vi "akcelerometr.vi"() -> ()   [LabVIEW 2014]
doc: "This example demonstrates how to read X, Y, and Z accelerations using the MMA8452 accelerometer."
uses:
  <vilib>/MakerHub/LINX/Public/Utilities/Open Local.vi
  <vilib>/MakerHub/LINX/LMH-LINX.lvlib
panel:
  out "k¹t nachylenia":dbl
  in  "Stop Button":bool
  out "Waveform Chart":T1(graph)
  out "Loop Rate (Hz)":u32
  # "LIS3DH Accelerometer\n\nThis example demonstrates how to read three axis of acceleration from the LIS3DH \\ MMA8452Q accelerometer \n\nInstructions\n1. Select the COM Port associated with the LINX Device.\n2. Select the I2C Channel that the MMA8452Q is connected to.\n3. Click the Run Arrow."
  # "Analog Value"
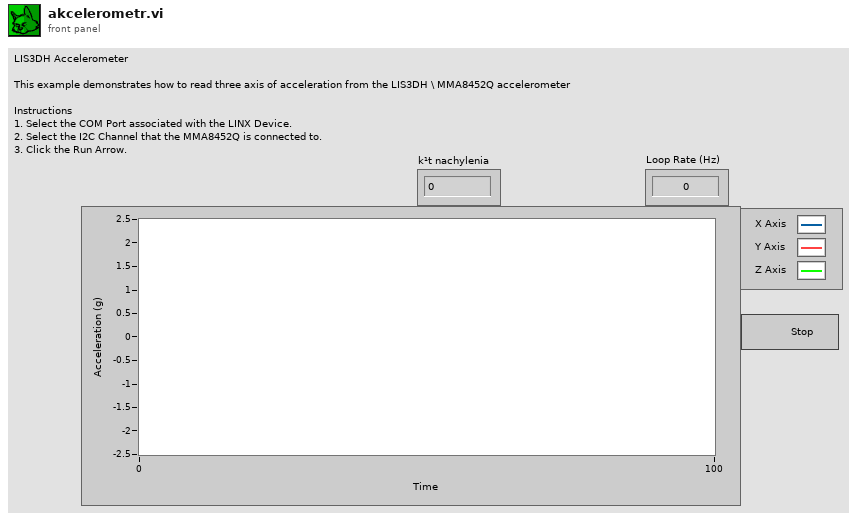
[diagram p1: front panel]
types:
  T1 = cluster{"X Axis":dbl, "Y Axis":dbl, "Z Axis":dbl}
  T2 = typedef "LMH-LINX.lvlib/LINX Ref.ctl" = cluster{"IO":T3, "Interface":T4, "LINX Device Config":T5}
  T3 = typedef "LMH-LINX.lvlib/Platform.ctl" = enum16{"Remote", "Local"}
  T4 = typedef "LMH-LINX.lvlib/Interface.ctl" = enum16{"Serial", "TCP"}
  T5 = typedef "LMH-LINX.lvlib/Device.lvlib/LINX Device Config.ctl" = cluster{"Interface":T4, "COM Port":refnum<visa-resource-name>, "TCP Configuration":T6, "Device Family":u8, "Device ID":u8, "Device Name":string, "TCP Ref":refnum<k5>, "Channels":T7}
  T6 = typedef "LMH-LINX.lvlib/Device.lvlib/TCP Config.ctl" = cluster{"IP Address":string, "Port":u16}
  T7 = typedef "LMH-LINX.lvlib/Channels.ctl" = cluster{"DI":u8[], "DO":u8[], "AI":u8[], "AO":u8[], "PWM":u8[], "QE":u8[], "UART":u8[], "I2C 2":u8[], "SPI":u8[], "CAN":u8[], "Servo":u8[], "AI Ref (V)":dbl, "AI Resolution (Bits)":u8, "AO Ref (V)":dbl, "AO Resolution (Bits)":u8}
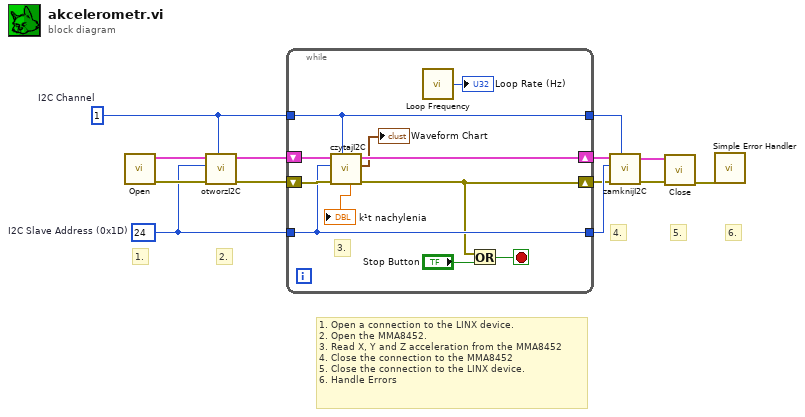
[diagram p0: block diagram]
diagram:
  w8 = u8 1  # I2C Channel
  w7 = u8 24  # I2C Slave Address (0x1D)
  # "6."
  # "4."
  # "2."
  # "5."
  # "1. Open a connection to the LINX device.\n2. Open the MMA8452.\n3. Read X, Y and Z acceleration from the MMA8452\n4. Close the connection to the MMA8452\n5. Close the connection to the LINX device.\n6. Handle Errors"
  # "1."
  n1 = call-poly <vilib>:"Open.vi"() -> ("Error Out"=w12:errorcluster, "LINX Resource"=w9:T2)  [unwired: 9 in, 1 out]
  n2 = call "otworzI2C.vi"("I2C Channel"=w8, "Error In"=w12, "I2C Slave Address (0x1D)"=w7, "LINX Ref"=w9) -> ("Error Out"=w11:errorcluster, "LINX Resource"=w10:T2)  [unwired: 6 in]
  n3 = while {
    tunnel: w8 -> [w18]
    tunnel: w7 -> [w20]
    shift-right: [w17] -> w1
    shift-left: w10 -> [w19]
    shift-right: [w16] -> w5
    shift-left: w11 -> [w21]
    tunnel: [w18] -> w2
    tunnel: [w20] -> w6
    stop <- w23 stop-if-true
    # "3."
    n4 = call "czytajI2C.vi"("I2C Channel"=w18, "Error In"=w21, "I2C Slave Address (0x1D)"=w20, "LINX Resource in"=w19) -> ("Error Out"=w16:errorcluster, "Acceleration Data (g)"=→"Waveform Chart":T1, "LINX Resource out"=w17:T2, "k¹t nachylenia"=→"k¹t nachylenia":dbl)  [unwired: 3 in, 1 out]
    n5 = call <vilib>:"Loop Frequency.vi"() -> ("Loop Rate (Hz)"=→"Loop Rate (Hz)":u32)
    n6 = Or(x=w16, y="Stop Button") -> (x .or. y?=w23:bool)
  }
  n7 = call "zamknijI2C.vi"("I2C Channel (0)"=w2, "Error In"=w5, "I2C Slave Address (0)"=w6, "LINX Resource"=w1) -> ("Error Out"=w4:errorcluster, "LINX Resource"=w3:T2)  [unwired: 6 in]
  n8 = call <vilib>:"Close.vi"("Error In"=w4, "LINX Resource"=w3) -> ("Error Out"=w13:errorcluster)  [unwired: 9 in]
  n9 = call <vilib>:"Simple Error Handler.vi"("error in (no error)"=w13) -> ()  [unwired: 4 in, 5 out]
